vi "Init Phidget servos.vi"() -> (1 "Device Out":i32, 2 "Engaged?":bool, 3 "error out":errorcluster)   [LabVIEW 2014]
doc: "This VI will initalize the servos for the Act laser pointing device."
panel:
  out "Serial Number Return":i32
  out "Number of\nservos":i32
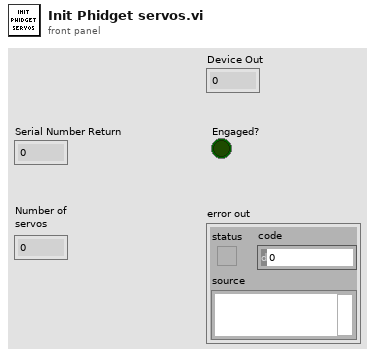
[diagram p1: front panel]
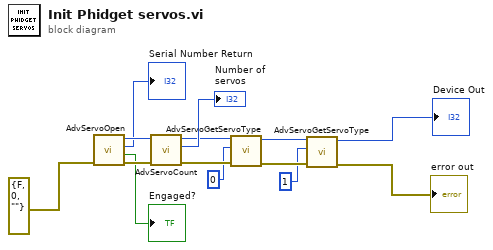
[diagram p0: block diagram]
diagram:
  n1 = call "AdvServoOpen.vi"("error in"=errorcluster {"status"=FALSE, "code"=0, "source"=""} ("error in (no error)")) -> ("error out"=w13:errorcluster, "Attached?"=→"Engaged?":bool, "Serial Number Return"=→"Serial Number Return":i32, "Device Out"=w12:i32)  [unwired: 7 in]
  n2 = call "AdvServoCount.vi"("error in (no error)"=w13, "Device In"=w12) -> ("error out"=w7:errorcluster, "count"=→"Number of\nservos":i32, "Device Out"=w8:i32)  [unwired: 7 in]
  n3 = call "AdvServoGetServoType.vi"("error in (no error)"=w7, "index"=0, "Device In"=w8) -> ("error out"=w4:errorcluster, "Device Out"=w5:i32)  [unwired: 5 in, 1 out]
  n4 = call "AdvServoGetServoType.vi"("error in (no error)"=w4, "index"=1, "Device In"=w5) -> ("error out"=→"error out":errorcluster, "Device Out"=→"Device Out":i32)  [unwired: 5 in, 1 out]
